vi "Line Search Prep (VI).vi"(6 "data":variant, 7 "F(X)":T2, 8 "TOLX":dbl=1e-07, 9 "P":dbl[](array[numeric]), 10 "X":dbl[](array[numeric]), 11 "J":T1) -> (0 "error":i32, 1 "F(X)*F(X)":dbl, 2 "tolerance":dbl, 3 "X * Y":dbl)   [LabVIEW 2020, in "NI_Gmath.lvlib"]
uses:
  NI_Gmath.lvlib
  functionRefnum nD.ctl
  RealMatrix.ctl
  Real Dot Product.vi
  A x Vector.vi
  NI_AALBase.lvlib
  NI_Matrix.lvlib
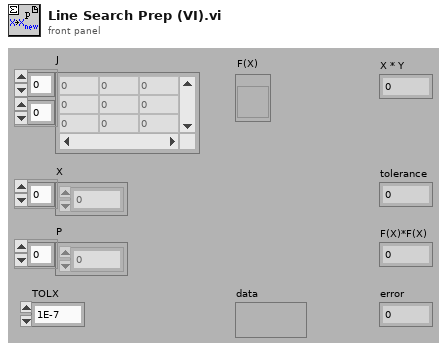
[diagram p1: front panel]
types:
  T1 = typedef "NI_Matrix.lvlib/RealMatrix.ctl" = dbl[][]
  T2 = typedef "NI_Gmath.lvlib/functionRefnum nD.ctl" = refnum<vi>
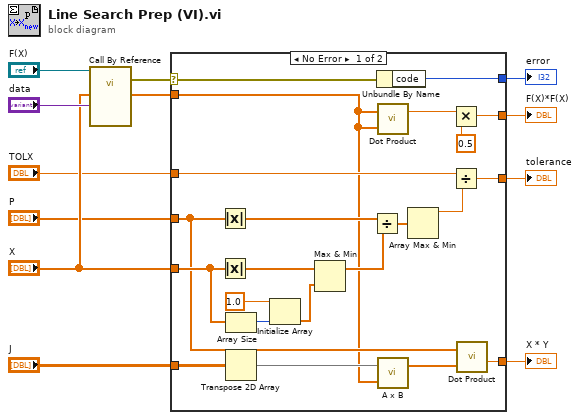
[diagram p0: block diagram]
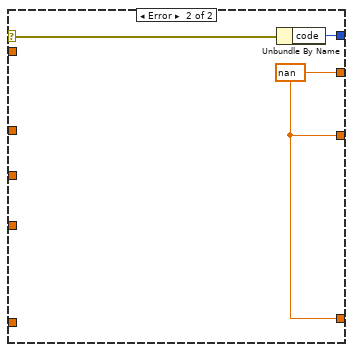
[diagram p2: hidden frame]
diagram:
  n1 = call-by-ref "?"(reference="F(X)", "variant"="data", "X"="X") -> (error out=w2:errorcluster, "F(X)"=w10:dbl[])  [unwired: 4 in, 1 out]
  n2 = case shown="No Error" w2 {
    selector: w2 -> [w16 w37]
    tunnel: w10 -> [w14 _]
    tunnel: [w23 w35] -> w9
    tunnel: [w22 w35] -> w8
    tunnel: [w21 w35] -> w7
    tunnel: "X" -> [w20 _]
    tunnel: "TOLX" -> [w19 _]
    tunnel: "J" -> [w18 _]
    tunnel: "P" -> [w17 _]
    tunnel: [w15 w36] -> w1
    frame No Error {
      n3 = Absolute Value(x=w17) -> (abs(x)=w30:dbl[])
      n4 = Absolute Value(x=w20) -> (abs(x)=w29:dbl[])
      n5 = Array Size(array=w20) -> (size(s)=w27:i32)
      n6 = Transpose 2D Array(2D array=w18) -> (transposed array=w24:T1)
      n7 = Initialize Array(1.0, w27) -> (w28:dbl[])
      n8 = Max & Min(x=w29, y=w28) -> (max(x,y)=w31:dbl[])  [unwired: 1 out]
      n9 = Divide(x=w30, y=w31) -> (x/y=w32:dbl[])
      n10 = Unbundle By Name(w16) -> ("code"=w15:i32)
      n11 = call-poly "Dot Product.vi"("Y Vector"=w14, "X Vector"=w14) -> ("X * Y"=w13:dbl)  [unwired: 1 out]
      n12 = call-poly "A x B.vi"("Vector"=w14, "A"=w24) -> ("A x Vector"=w25:dbl[])  [unwired: 1 out]
      n13 = Array Max & Min(array=w32) -> (max value=w33:dbl)  [unwired: 3 out]
      n14 = Multiply(x=w13, y=0.5) -> (x*y=w23:dbl)
      n15 = Divide(x=w19, y=w33) -> (x/y=w22:dbl)
      n16 = call-poly "Dot Product.vi"("Y Vector"=w25, "X Vector"=w17) -> ("X * Y"=w21:dbl)  [unwired: 1 out]
    }
    frame Error {
      w35 = nan
      n17 = Unbundle By Name(w37) -> ("code"=w36:i32)
    }
  }
  "error" <- w1
  "X * Y" <- w7
  "tolerance" <- w8
  "F(X)*F(X)" <- w9
